vi "Blink.vi"() -> ()   [LabVIEW 2014]
uses:
  <userlib>/UCSD Robotics Lab/Robotics-Cape/LV/libroboticscape.lvlib
panel:
  out "Timing Block":T1 {"Actual Hz" format="%#_3g"; "Dt" format="%#_4g"; "Average Hz" format="%#_4g"}
  out "Mode":dbl
  out "State":T2(ring)
  in  "stop":bool
  # "Always stop the VI using the rectangular STOP button above, never with the round stopsign (Abort)"
  # "Press mode button to change blink rate\nHold Pause button to exit\nPress and release Pause button to pause"
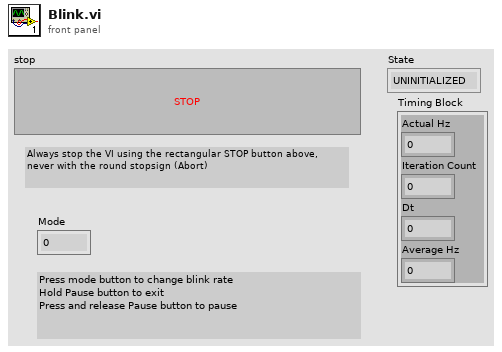
[diagram p1: front panel]
types:
  T1 = cluster{"Actual Hz":dbl, "Iteration Count":dbl, "Dt":dbl, "Average Hz":dbl}
  T2 = enum16{"UNINITIALIZED", "RUNNING", "PAUSED", "EXITING"}
  T3 = cluster{"Pause Press Event":refnum<user-event>, "Pause Release Event":refnum<user-event>, "Mode Press Event":refnum<user-event>, "Mode Release Event":refnum<user-event>}
  T4 = enum16{"UNINITIALIZED", "RUNING", "PAUSED", "EXITING"}
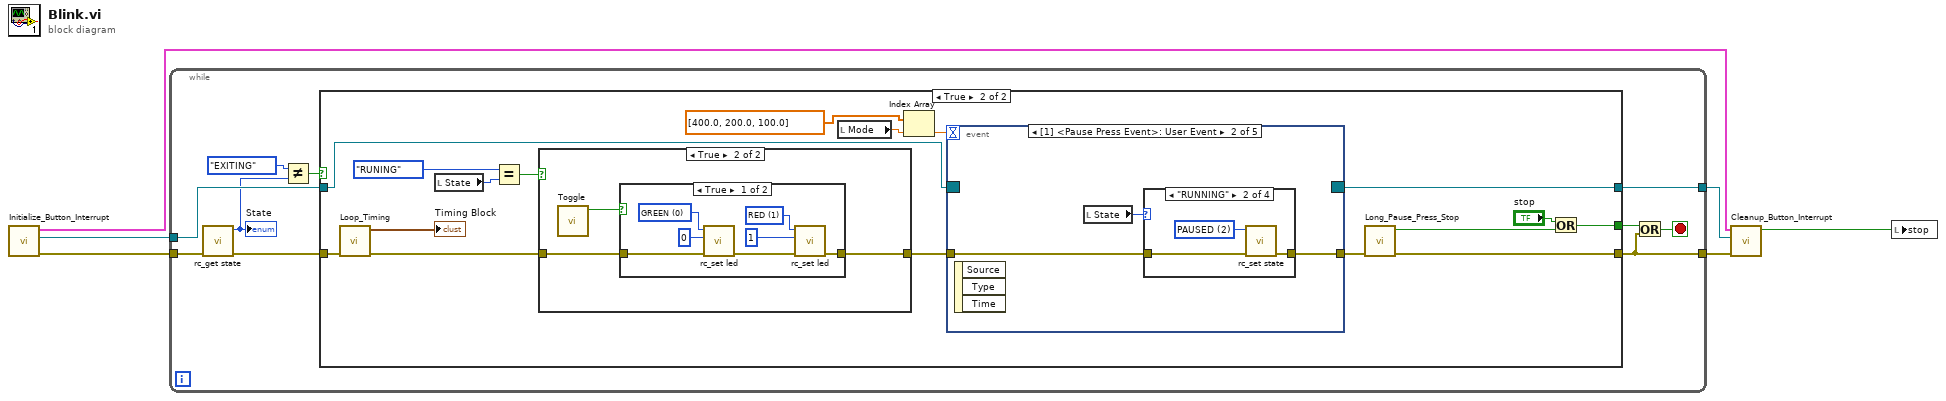
[diagram p0: block diagram]
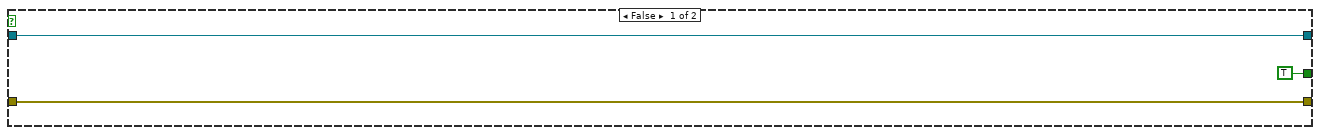
[diagram p2: hidden frame]
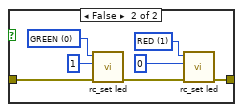
[diagram p4: hidden frame]
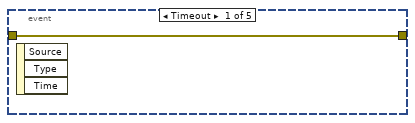
[diagram p5: hidden frame]
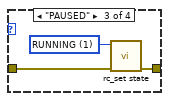
[diagram p7: hidden frame]
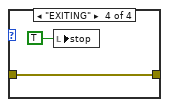
[diagram p8: hidden frame]
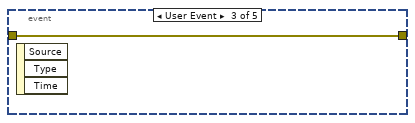
[diagram p9: hidden frame]
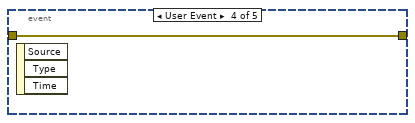
[diagram p10: hidden frame]
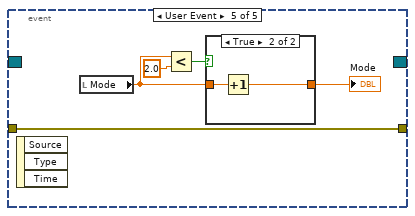
[diagram p11: hidden frame]
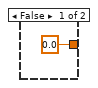
[diagram p12: hidden frame]
diagram:
  n1 = call "Initialize_Button_Interrupt.vi"() -> ("error out"=w6:errorcluster, "Event Registration Refnum 2"=w1:refnum<event-registration>, "Button Events"=w3:T3)  [unwired: 9 in]
  n2 = while {
    tunnel: w6 -> [w15]
    tunnel: [w11] -> w4
    tunnel: [w8] -> w2
    tunnel: w1 -> [w9]
    stop <- w16 stop-if-true
    n3 = call <userlib>:"rc_get state.vi"("error in (no error)"=w15) -> ("error out"=w12:errorcluster, "function return"=w7:u32)  [unwired: 9 in]
    "State" <- w7
    n4 = Not Equal?(x=T4."EXITING" ("State 2"), y=w7) -> (x != y?=w13:bool)
    n5 = case shown="True" w13 {
      tunnel: w12 -> [w19 w27]
      tunnel: [w19 w23] -> w11
      tunnel: [TRUE ("stop") w20] -> w10
      tunnel: w9 -> [w17 w36]
      tunnel: [w17 w35] -> w8
      frame False {
      }
      frame True {
        n6 = call "Loop_Timing.vi"("error in"=w27) -> ("error out"=w26:errorcluster, "Timing Block"=→"Timing Block":T1)  [unwired: 9 in]
        n7 = local read "State"() -> (w29:T2)
        n8 = Equal?(x=T4."RUNING" ("State 2"), y=w29) -> (x = y?=w31:bool)
        n9 = case shown="True" w31 {
          tunnel: w26 -> [w37 w39]
          tunnel: [w37 w38] -> w34
          frame False {
          }
          frame True {
            n10 = call "Toggle.vi"() -> ("Boolean"=w40:bool)  [unwired: 11 in]
            n11 = case shown="True" w40 {
              tunnel: w39 -> [w47 w54]
              tunnel: [w41 w52] -> w38
              frame True {
                w44 = u32 1 items=["GREEN", "RED"] ("led")
                w45 = u32 0 items=["GREEN", "RED"] ("led")
                n12 = call <userlib>:"rc_set led.vi"("error in (no error)"=w47, "state"=0, "led"=w45) -> ("error out"=w46:errorcluster)  [unwired: 7 in, 1 out]
                n13 = call <userlib>:"rc_set led.vi"("error in (no error)"=w46, "state"=1, "led"=w44) -> ("error out"=w41:errorcluster)  [unwired: 7 in, 1 out]
              }
              frame False {
                w50 = u32 1 items=["GREEN", "RED"] ("led")
                w51 = u32 0 items=["GREEN", "RED"] ("led")
                n14 = call <userlib>:"rc_set led.vi"("error in (no error)"=w54, "state"=1, "led"=w51) -> ("error out"=w53:errorcluster)  [unwired: 7 in, 1 out]
                n15 = call <userlib>:"rc_set led.vi"("error in (no error)"=w53, "state"=0, "led"=w50) -> ("error out"=w52:errorcluster)  [unwired: 7 in, 1 out]
              }
            }
          }
        }
        n16 = local read "Mode"() -> (w33:dbl)
        n17 = Index Array(array=dbl[] [400.0, 200.0, 100.0], index=w33) -> (element=w28:dbl)
        n18 = event shown="[1] <Pause Press Event>: User Event" {
          selector: w36 -> [_ _ _ _ _]
          dyn-events: [_ _ _ _ _] -> w35
          timeout: w28 -> [_ _ _ _ _]
          tunnel: w34 -> [w55 w58 w68 w69 w74]
          tunnel: [w55 w56 w68 w69 w74] -> w24
          event Timeout {
            n19 = event-data() -> ()  [unwired: 1 in, 3 out]
          }
          event User Event {
            n20 = event-data() -> ()  [unwired: 1 in, 3 out]
            n21 = local read "State"() -> (w57:T2)
            n22 = case shown="\"RUNNING\"" w57 {
              tunnel: w58 -> [w59 w62 w65 w67]
              tunnel: [w59 w61 w64 w67] -> w56
              frame "UNINITIALIZED", Default {
              }
              frame "RUNNING" {
                w60 = u32 2 items=["UNINITIALIZED", "RUNNING", "PAUSED", "EXITING"] ("new_state")
                n23 = call <userlib>:"rc_set state.vi"("error in (no error)"=w62, "new_state"=w60) -> ("error out"=w61:errorcluster)  [unwired: 8 in, 1 out]
              }
              frame "PAUSED" {
                w63 = u32 1 items=["UNINITIALIZED", "RUNNING", "PAUSED", "EXITING"] ("new_state")
                n24 = call <userlib>:"rc_set state.vi"("error in (no error)"=w65, "new_state"=w63) -> ("error out"=w64:errorcluster)  [unwired: 8 in, 1 out]
              }
              frame "EXITING" {
                n25 = local write "stop"(TRUE ("stop")) -> ()
              }
            }
          }
          event User Event {
            n26 = event-data() -> ()  [unwired: 1 in, 3 out]
          }
          event User Event {
            n27 = event-data() -> ()  [unwired: 1 in, 3 out]
          }
          event User Event {
            n28 = event-data() -> ()  [unwired: 1 in, 3 out]
            n29 = local read "Mode"() -> (w72:dbl)
            n30 = Less?(x=w72, y=2.0) -> (x < y?=w70:bool)
            n31 = case shown="True" w70 {
              tunnel: w72 -> [_ w77]
              tunnel: [0.0 w76] -> w73
              frame False {
              }
              frame True {
                n32 = Increment(x=w77) -> (x+1=w76:dbl)
              }
            }
            "Mode" <- w73
          }
        }
        n33 = call "Long_Pause_Press_Stop.vi"("error in (no error)"=w24) -> ("error out"=w23:errorcluster, "Stop"=w21:bool)  [unwired: 9 in]
        n34 = Or(x="stop", y=w21) -> (x .or. y?=w20:bool)
      }
    }
    n35 = Or(x=w10, y=w11) -> (x .or. y?=w16:bool)
  }
  n36 = call "Cleanup_Button_Interrupt.vi"("error in (no error)"=w4, "Event Registration Refnum"=w2, "Button Events"=w3) -> ("Stop Local Variabl"=w5:bool)  [unwired: 6 in]
  n37 = local write "stop"(w5) -> ()
